vi "Log Response.vi"(9 "Acknowledge Data":T1, 10 "Module Action":string, 11 "Module Data In":refnum<class "Rename.lvclass">) -> (0 "error out":errorcluster, 3 "Module Data Out":refnum<class "Rename.lvclass">)   [LabVIEW 2015, in "Generic Module Library.lvlib" / "Template G_Module.lvlib"]
uses:
  Template G_Module.lvlib
  Module Class/Rename.lvclass
  Private Controls/Module Message Cluster Components/Acknowledge Data Cluster.ctl
  Private Controls/Module Message Cluster Components/Ack Payload.ctl
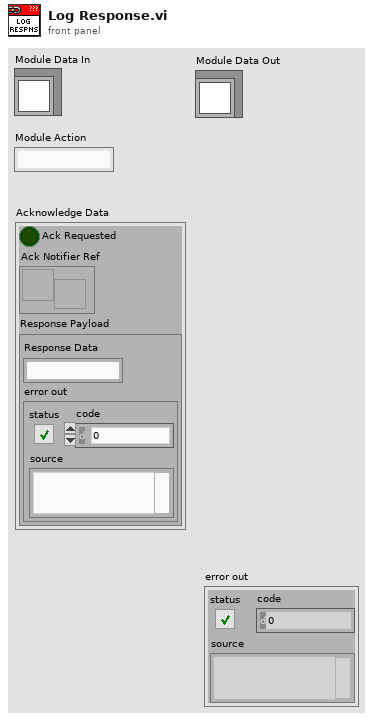
[diagram p1: front panel]
types:
  T1 = typedef "Generic Module Library.lvlib/Template G_Module.lvlib/Acknowledge Data Cluster.ctl" = cluster{"Ack Requested":bool, "Ack Notifier Ref":refnum<notifier>, "Response Payload":T2}
  T2 = typedef "Generic Module Library.lvlib/Template G_Module.lvlib/Ack Payload.ctl" = cluster{"Response Data":string, "error out":errorcluster}
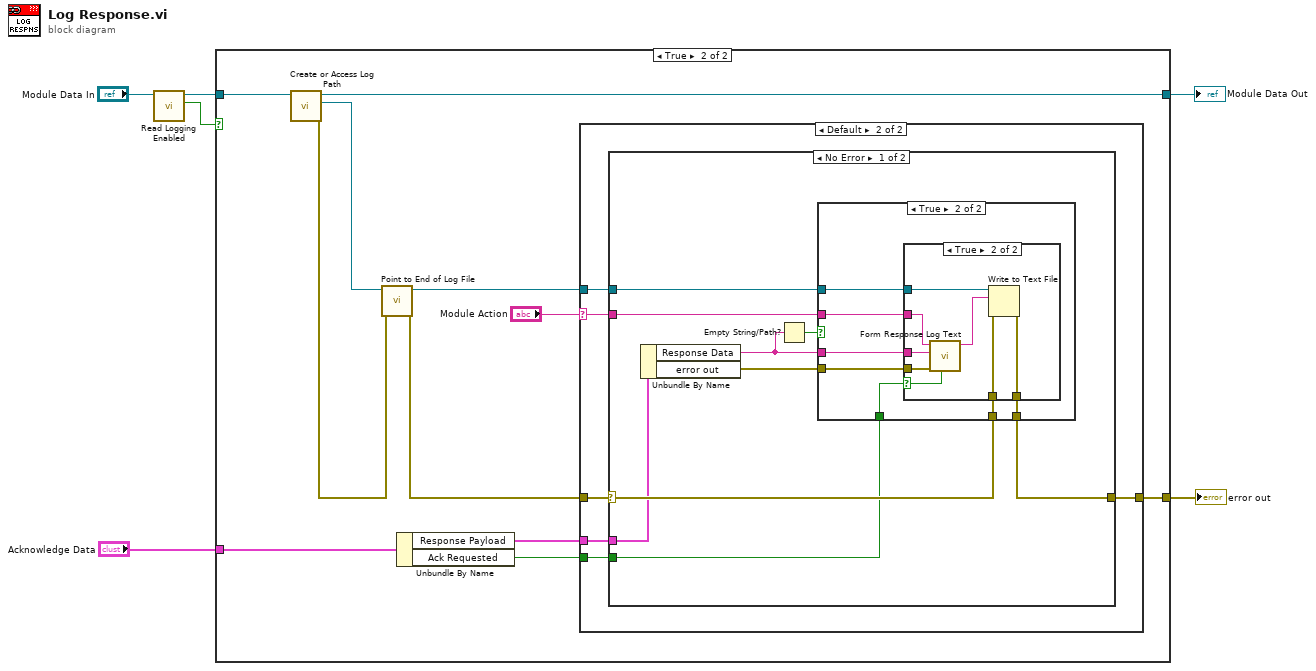
[diagram p0: block diagram]
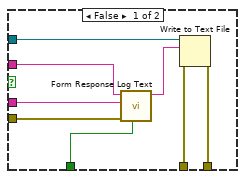
[diagram p4: hidden frame]
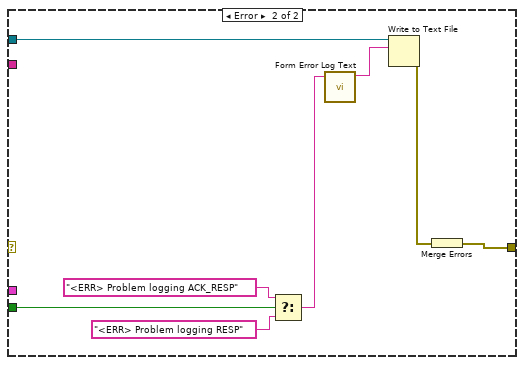
[diagram p6: hidden frame]
diagram:
  n1 = call-dynamic "Read Logging Enabled.vi"("Rename in"="Module Data In") -> ("Logging Enabled"=w2:bool, "Rename out"=w3:refnum<class "Rename.lvclass">)  [unwired: 8 in, 1 out]
  n2 = case shown="True" w2 {
    tunnel: w3 -> [w7 w18]
    tunnel: [_ w16] -> w6
    tunnel: "Acknowledge Data" -> [_ w15]
    tunnel: [w7 w8] -> w1
    frame False {
    }
    frame True {
      n3 = call "Create or Access Log Path.vi"("Module Data In"=w18) -> ("error out"=w14:errorcluster, "Log Refnum Out"=w17:refnum<file>, "Module Data Out"=w8:refnum<class "Rename.lvclass">)  [unwired: 7 in, 1 out]
      n4 = call "Point to End of Log File.vi"("error in (no error)"=w14, "Byte Stream File in"=w17) -> ("error out"=w12:errorcluster, "Byte Stream File out"=w13:refnum<file>)  [unwired: 8 in]
      n5 = Unbundle By Name(w15) -> ("Response Payload"=w10:T2, "Ack Requested"=w11:bool)
      n6 = case shown="Default" "Module Action" {
        selector: "Module Action" -> [_ w20]
        tunnel: [w19 w25] -> w16
        tunnel: w13 -> [_ w24]
        tunnel: w12 -> [w19 w23]
        tunnel: w11 -> [_ w22]
        tunnel: w10 -> [_ w21]
        frame "Timeout" {
        }
        frame Default {
          n7 = case shown="No Error" w23 {
            selector: w23 -> [w32 _]
            tunnel: w24 -> [w31 w63]
            tunnel: [w34 w66] -> w25
            tunnel: w21 -> [w27 _]
            tunnel: w20 -> [w33 _]
            tunnel: w22 -> [w30 w61]
            frame No Error {
              n8 = Unbundle By Name(w27) -> ("Response Data"=w29:string, "error out"=w26:errorcluster)
              n9 = Empty String/Path?(string/path=w29) -> (empty?=w28:bool)
              n10 = case shown="True" w28 {
                tunnel: [w42 w47] -> w34
                tunnel: w33 -> [w41 w43]
                tunnel: w29 -> [w40 w45]
                tunnel: w32 -> [w39 w48]
                tunnel: w31 -> [w38 w46]
                tunnel: w30 -> [w36 w49]
                tunnel: w26 -> [w35 w44]
                frame False {
                  n11 = call "Form Response Log Text.vi"("ACK"=w36, "error in"=w35, "Ack Data Input"=w40, "Module Action"=w41) -> ("String to Write"=w37:string)  [unwired: 7 in]
                  n12 = Write to Text File(file (use dialog)=w38, text=w37, error in=w39) -> (error out=w42:errorcluster)  [unwired: 1 in, 2 out]
                }
                frame True {
                  n13 = case shown="True" w49 {
                    selector: w49 -> [_ w53]
                    tunnel: w48 -> [w50 w57]
                    tunnel: [w50 w56] -> w47
                    tunnel: w46 -> [_ w58]
                    tunnel: w43 -> [_ w55]
                    tunnel: w45 -> [_ w52]
                    tunnel: w44 -> [_ w51]
                    frame False {
                    }
                    frame True {
                      n14 = call "Form Response Log Text.vi"("ACK"=w53, "error in"=w51, "Ack Data Input"=w52, "Module Action"=w55) -> ("String to Write"=w54:string)  [unwired: 7 in]
                      n15 = Write to Text File(file (use dialog)=w58, text=w54, error in=w57) -> (error out=w56:errorcluster)  [unwired: 1 in, 2 out]
                    }
                  }
                }
              }
            }
            frame Error {
              n16 = Select(t="<ERR> Problem logging ACK_RESP" ("Error Source Input"), s=w61, f="<ERR> Problem logging RESP") -> (s? t:f=w59:string)
              n17 = call "Form Error Log Text.vi"("Error Source Input"=w59) -> ("String to Write"=w64:string)  [unwired: 10 in]
              n18 = Write to Text File(file (use dialog)=w63, text=w64) -> (error out=w65:errorcluster)  [unwired: 2 in, 2 out]
              n19 = Merge Errors(w65) -> (w66:errorcluster)
            }
          }
        }
      }
    }
  }
  "error out" <- w6
  "Module Data Out" <- w1
